vi "Variant_to_Waveform_info.vi"(8 "Error in":errorcluster, 11 "Value (in)":variant) -> (0 "Error out":errorcluster, 2 "Value (string)":string, 3 "Value (out)":waveform(dbl))   [LabVIEW 2012]
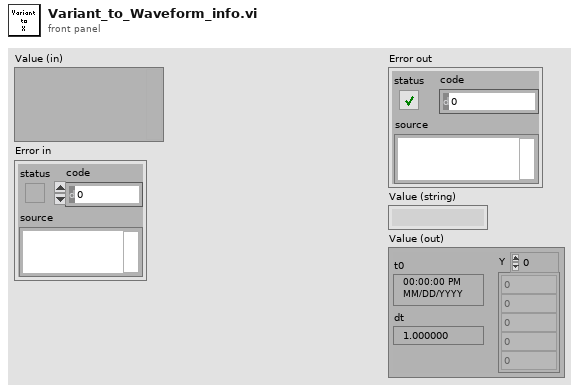
[diagram p1: front panel]
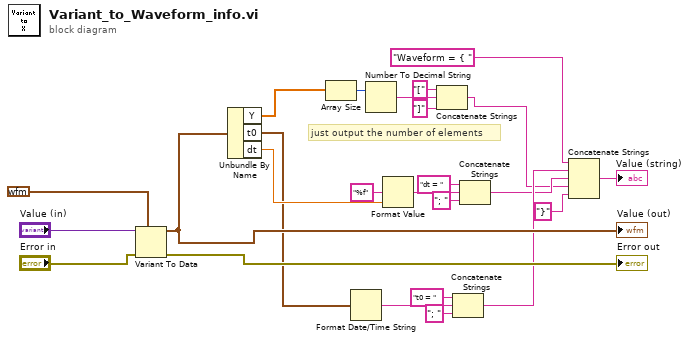
[diagram p0: block diagram]
diagram:
  # "just output the number of elements"
  n1 = Variant To Data(error in="Error in", type=waveform(dbl) {"t0"=timestamp(0 s since 1904-01-01), "dt"=1.0, "Y"=[]} ("Waveform"), Variant="Value (in)") -> (data=w22:waveform(dbl), error out=→"Error out":errorcluster)
  "Value (out)" <- w22
  n2 = Unbundle By Name(w22) -> ("Y"=w20:dbl[], "t0"=w14:timestamp, "dt"=w18:dbl)
  n3 = Array Size(array=w20) -> (size(s)=w6:i32)
  n4 = Format Date/Time String(seconds (now)=w14) -> (date/time string=w11:string)  [unwired: 2 in]
  n5 = Number To Decimal String(number=w6) -> (decimal integer string=w5:string)  [unwired: 1 in]
  n6 = Format Value(format string="%f", value (0)=w18) -> (output string=w17:string)  [unwired: 1 in]
  n7 = Concatenate Strings("[" ("string"), w5, "]" ("string")) -> (w8:string)
  n8 = Concatenate Strings("t0 = " ("string"), w11, "; " ("string")) -> (w10:string)
  n9 = Concatenate Strings("dt = " ("string"), w17, "; " ("string")) -> (w9:string)
  n10 = Concatenate Strings("Waveform = { " ("string"), w10, w9, w8, "}" ("string")) -> (→"Value (string)":string)
